vi "PlatMods to Zoom mods.vi"(11 "PlatMods":T2) -> (3 "ZoomMods":T1)   [LabVIEW 2021, in "RocketPlot.lvlib"]
uses:
  RocketPlot.lvlib
  TypeDefs/ZoomCache PlatMod.ctl
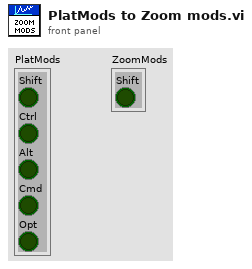
[diagram p1: front panel]
types:
  T1 = typedef "RocketPlot.lvlib/ZoomCache PlatMod.ctl" = cluster{"Shift":bool}
  T2 = cluster{"Shift":bool, "Ctrl":bool, "Alt":bool, "Cmd":bool, "Opt":bool}
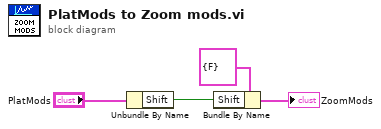
[diagram p0: block diagram]
diagram:
  n1 = Unbundle By Name("PlatMods") -> ("Shift"=w2:bool)
  n2 = Bundle By Name(cluster=T1 {"Shift"=FALSE} ("Cluster"), "Shift"=w2) -> (→"ZoomMods":T1)
